vi "Set Ring Exposure Times.vi"(10 "times":sgl, 11 "numTimes":i32) -> (2 "times out":sgl, 3 "function return":u32)   [LabVIEW 2018, in "AndorSDK.lvlib"]
doc: "EXPNETTYPE unsigned int WINAPI SetRingExposureTimes(int numTimes, float * times);"
uses:
  AndorSDK.lvlib
  ATMCD32D.dll
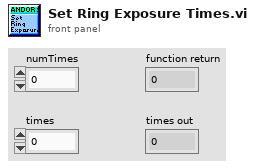
[diagram p1: front panel]
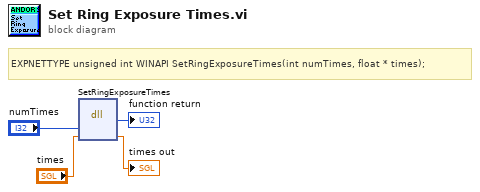
[diagram p0: block diagram]
diagram:
  # "EXPNETTYPE unsigned int WINAPI SetRingExposureTimes(int numTimes, float * times);"
  n1 = dll-call lib="PTH2babs E\nPersönliches02 - Arbeit03-HiwijobsLabviewCodelibANDOR\tAndor SDK\nATMCD32D.*" fn="SetRingExposureTimes"("numTimes"="numTimes", "times"="times") -> (→"function return":u32, "times"=→"times out":sgl)  [unwired: 4 in, 2 out]
